vi "TemperatureToError.vi"(0 "Temperature / C":dbl=25.0 format="%#_13g", 1 "Rgain":dbl=100000.0, 2 "Vref":dbl=1.0, 3 "Rset":dbl=10000.0, 4 "Polarity":bool=TRUE) -> (5 "Reading":dbl=1.726578555962758e-05, 6 "I":dbl=9.999956835536101e-05)   [LabVIEW 2014]
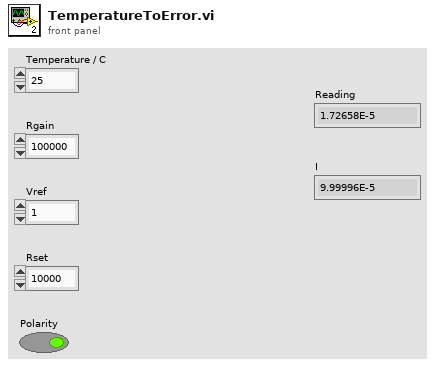
[diagram p1: front panel]
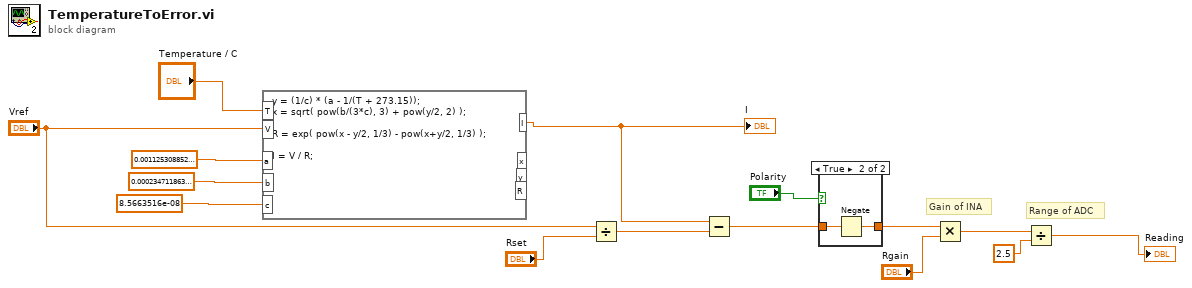
[diagram p0: block diagram]
diagram:
  # "Gain of INA"
  # "Range of ADC"
  n1 = formula code="y = (1/c) * (a - 1/(T + 273.15));\nx = sqrt( pow(b/(3*c), 3) + pow(y/2, 2) );\n\nR = exp( pow(x - y/2, 1/3) - pow(x+y/2, 1/3) );\n\nI = V / R;"("a"=0.001125308852122, "b"=0.000234711863267, "c"=8.5663516e-08, "T"="Temperature / C", "V"="Vref") -> ("I"=w8:dbl)  [unwired: 3 out]
  "I" <- w8
  n2 = Divide(x="Vref", y="Rset") -> (x/y=w9:dbl)
  n3 = Subtract(x=w8, y=w9) -> (x-y=w7:dbl)
  n4 = case shown="True" "Polarity" {
    tunnel: w7 -> [w16 w18]
    tunnel: [w16 w17] -> w2
    frame False {
    }
    frame True {
      n5 = Negate(x=w18) -> (-x=w17:dbl)
    }
  }
  n6 = Multiply(x=w2, y="Rgain") -> (x*y=w4:dbl)
  n7 = Divide(x=w4, y=2.5) -> (x/y=→"Reading":dbl)
